vi "Find Subkeys.vi"(9 "Full Path? (false)":bool, 10 "Keys":string[](array[string]), 11 "Key Root":string) -> (2 "Subkeys":string[](array[string]))   [LabVIEW 2019]
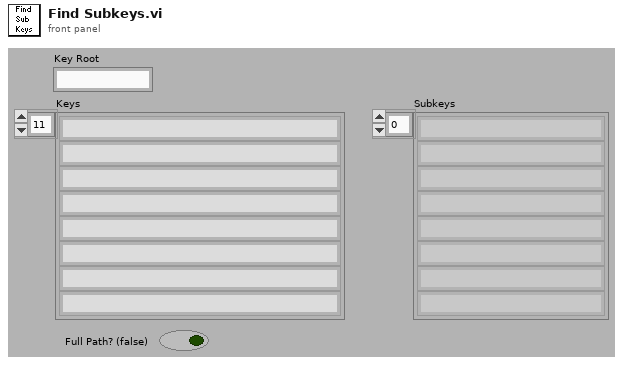
[diagram p1: front panel]
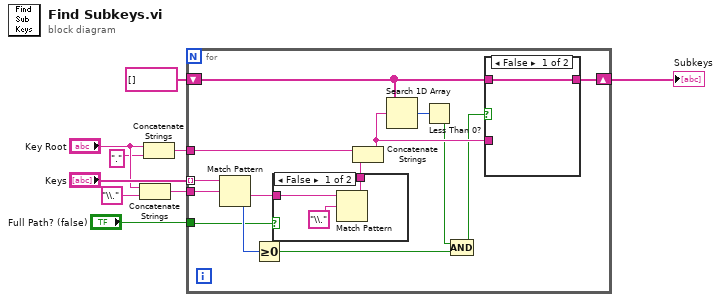
[diagram p0: block diagram]
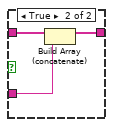
[diagram p3: hidden frame]
diagram:
  n1 = Concatenate Strings("Key Root", "\\." ("string")) -> (w8:string)
  n2 = Concatenate Strings("Key Root", "." ("string")) -> (w3:string)
  n3 = for {
    tunnel: "Keys" -> [w23] mode=indexing
    tunnel: w8 -> [w21]
    shift-right: [w20] -> w6
    shift-left: string[] [] -> [w17]
    tunnel: w3 -> [w11]
    tunnel: "Full Path? (false)" -> [w10]
    n4 = Match Pattern(string=w23, regular expression=w21) -> (after substring=w22:string, offset past match=w19:i32)  [unwired: 1 in, 2 out]
    n5 = Greater Or Equal To 0?(x=w19) -> (x >= 0?=w13:bool)
    n6 = case shown="False" w10 {
      tunnel: w22 -> [w26 w27]
      tunnel: [w24 w27] -> w18
      frame False {
        n7 = Match Pattern(string=w26, regular expression="\\.") -> (before substring=w24:string)  [unwired: 1 in, 3 out]
      }
      frame True {
      }
    }
    n8 = Concatenate Strings(w11, w18) -> (w16:string)
    n9 = Search 1D Array(1D array=w17, element=w16) -> (index of element=w15:i32)  [unwired: 1 in]
    n10 = Less Than 0?(x=w15) -> (x < 0?=w12:bool)
    n11 = Compound Arithmetic op=AND(w12, w13) -> (w14:bool)
    n12 = case shown="False" w14 {
      tunnel: [w28 w31] -> w20
      tunnel: w17 -> [w28 w30]
      tunnel: w16 -> [_ w29]
      frame False {
      }
      frame True {
        n13 = Build Array (concatenate)(w30, w29) -> (w31:string[])
      }
    }
  }
  "Subkeys" <- w6
